vi "MPVSenden_ECD.vi"(3 "Ventilposition":i32=1 min=1 max=6 step=1, 4 "error in":errorcluster, 5 "FPGA-VI-Referenz (Ausgang) 2":refnum<k20>) -> (0 "Ventilposition":i32, 1 "error out":errorcluster, 2 "FPGA-VI-Referenz (Ausgang)":refnum<k20>)   [LabVIEW 2017]
uses:
  GVVentilposition_ECD.vi
  GVZwischenspeicher.vi
  <vilib>/Utility/error.llb/Error Cluster From Error Code.vi
  <vilib>/rvi/errors/niLvFpgaAdjustHostInterfaceError.vi
  <vilib>/rvi/interface/nirviMethod/nirviMethod.xnode
  FPGA Bitfiles/HAGAR-V_FPGATargetECD_FPGA-ProgrammECD_LbBtUh8SPQY.lvbitx
  FPGA_ECD/FPGA-Programm_ECD.vi
  <vilib>/FPGAPlugInAG/cRIO-9035/niLvFpga_WriteFifo_cRIO-9035.vi
  <vilib>/rvi/errors/niLvFpgaMergeErrorWithErrorCode.vi
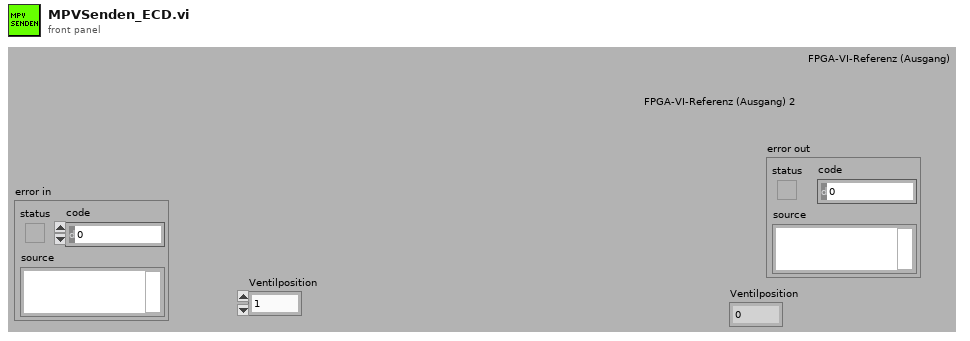
[diagram p1: front panel]
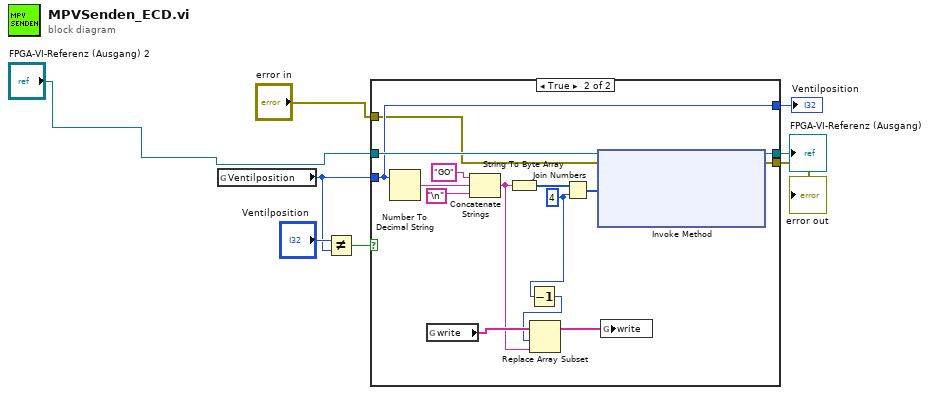
[diagram p0: block diagram]
diagram:
  n1 = global read "GVVentilposition_ECD.vi" "Ventilposition"() -> (w6:i32)
  n2 = Not Equal?(x="Ventilposition", y=w6) -> (x != y?=w7:bool)
  n3 = case shown="True" w7 {
    tunnel: "FPGA-VI-Referenz (Ausgang) 2" -> [w11 w26]
    tunnel: [w11 w20] -> w1
    tunnel: w6 -> [w10 w19]
    tunnel: [w10 w19] -> w5
    tunnel: "error in" -> [w9 w18]
    tunnel: [w9 w17] -> w3
    frame False {
    }
    frame True {
      w12 = u8 4
      n4 = Number To Decimal String(number=w19) -> (decimal integer string=w21:string)  [unwired: 1 in]
      n5 = global read "GVZwischenspeicher.vi" "write"() -> (w16:string[])
      n6 = Concatenate Strings("GO", w21, "\n") -> (w13:string)
      n7 = String To Byte Array(string=w13) -> (unsigned byte array=w24:u8[])
      n8 = Decrement(x=w12) -> (x-1=w14:u8)
      n9 = Replace Array Subset(array=w16, new element=w13, index=w14) -> (w15:string[])
      n10 = Join Numbers(hi=w24, lo=w12) -> ((hi.lo)=w23:u16[])
      n11 = xnode "Invoke Method"("FPGA-VI-Referenz (Eingang)"=w26, "Fehler (Eingang)"=w18, "Daten"=w23) -> ("FPGA-VI-Referenz (Ausgang)"=w20:refnum<k20>, "Fehler (Ausgang)"=w17:errorcluster)  [unwired: 1 in, 1 out]
      n12 = global write "GVZwischenspeicher.vi" "write"(w15) -> ()
    }
  }
  "Ventilposition" <- w5
  "error out" <- w3
  "FPGA-VI-Referenz (Ausgang)" <- w1
